vi "GT_CrdStatus.vi"(5 "rtn_In":cluster{"rtn":i16, "Func":string}, 6 "crd":i16, 7 "fifo":i16) -> (0 "rtn_Out":cluster{"rtn":i16, "Func":string}, 1 "fifo out":i16, 2 "crd out":i16, 3 "pSegment":i32, 4 "pRun":i16)   [LabVIEW 2014]
uses:
  VC6/gts.dll
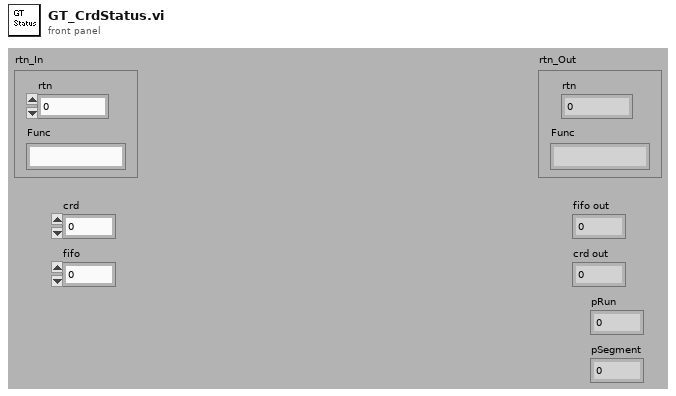
[diagram p1: front panel]
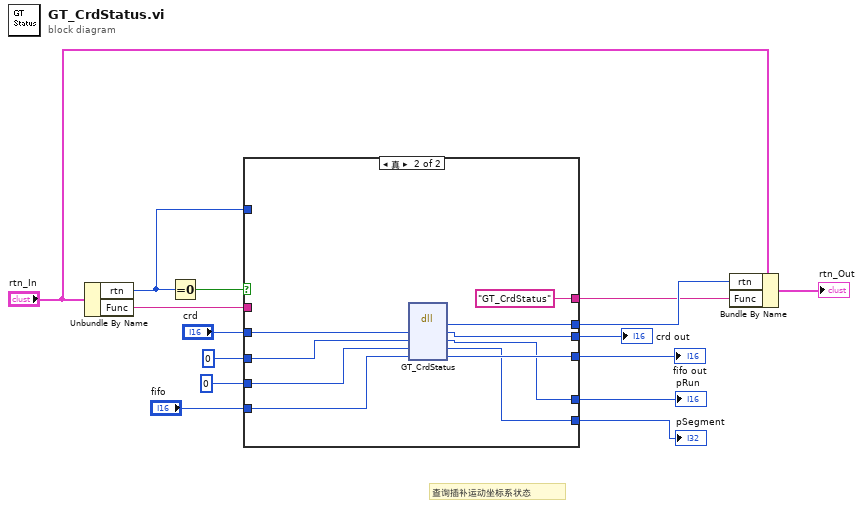
[diagram p0: block diagram]
diagram:
  # "查询插补运动坐标系状态"
  n1 = Unbundle By Name("rtn_In") -> ("rtn"=w3:i16, "Func"=w5:string)
  n2 = Equal To 0?(x=w3) -> (x = 0?=w15:bool)
  n3 = case shown="真" w15 {
    tunnel: [w20 w31] -> w12
    tunnel: [w21 "GT_CrdStatus" ("Func")] -> w11
    tunnel: "crd" -> [w19 w29]
    tunnel: i16 0 ("pRun") -> [w17 w28]
    tunnel: 0 ("pSegment") -> [w16 w27]
    tunnel: "fifo" -> [w18 w26]
    tunnel: [w18 w25] -> w6
    tunnel: w5 -> [w21 _]
    tunnel: [w19 w24] -> w4
    tunnel: w3 -> [w20 _]
    tunnel: [w17 w23] -> w2
    tunnel: [w16 w22] -> w1
    frame False {
    }
    frame True {
      n4 = dll-call lib="PTH2Fabs DNewGTS AC-800LWin7版源程序-20170926gts85VC6gts.dll" fn="GT_CrdStatus"("crd"=w29, "pRun"=w28, "pSegment"=w27, "fifo"=w26) -> ("rtn"=w31:i16, "crd"=w24:i16, "pRun"=w23:i16, "pSegment"=w22:i32, "fifo"=w25:i16)  [unwired: 3 in, 2 out]
    }
  }
  "fifo out" <- w6
  "crd out" <- w4
  "pRun" <- w2
  "pSegment" <- w1
  n5 = Bundle By Name(cluster="rtn_In", "rtn"=w12, "Func"=w11) -> (→"rtn_Out":cluster{"rtn":i16, "Func":string})
